vi "Dashboard Main.vi"() -> ()   [LabVIEW 2014]
uses:
  <vilib>/event_ctls.llb/eventvkey.ctl
  <vilib>/Rock Robotics/WPI/Dashboard/WPI_DashboardLogging Global.vi
  <vilib>/Utility/config.llb/Write Key (String).vi
  <vilib>/Utility/config.llb/Write Key (I32).vi
  <vilib>/Utility/config.llb/NI_LVConfig.lvlib
panel:
  out "Button 0":bool
  in  "TCP":refnum<k5>
  in  "Rec Mode":enum32{"Stop", "Record", "Playback"}(radio)
  in  "Vision":u16(ring) items=["Camera Off", "USB Camera SW", "USB Camera HW", "IP Camera"]
  out "Camera IP":string
  out "Image Message":string="Timeout in Camera Communications"
  in  "Dashboard Tab":T1(tab)
  in  "Camera Settings":T2={"Frame Rate"=30, "Compression"=30, "Size"=1} {"Frame Rate" scale=1.0..30.0; "Size" items=["640x480", "320x240", "160x120"]}
  out "MotorChart R":cluster{"Numeric":dbl, "Numeric":dbl}(graph)
  out "MotorChart L":T3(graph)
  out "MotorSliders R":cluster{"MotorSlide1":dbl, "MotorSlide2":dbl} {"MotorSlide2" scale=-1.0..1.0 scale format="%#_2e"; "MotorSlide1" scale=-1.0..1.0 scale format="%#_2e"}
  out "MotorSliders L":T4 {"MotorSlide4 2" scale=0.0..14.0 scale format="%#_2e"; "MotorSlide2" scale=-1.0..1.0 scale format="%#_2e"; "MotorSlide1" scale=-1.0..1.0 scale format="%#_2e"}
  out "Gyro":dbl(knob) scale=0.0..360.0
  out "JS1 Z":dbl(slide) scale=-1.0..1.0 scale format="%#_2e"
  out "JS1 Graph":cluster{"X":dbl, "Y":dbl}[](graph)
  out "JS1 Buttons":T5
  out "JS2 Z":dbl(slide) scale=-1.0..1.0 scale format="%#_2e"
  out "JS2 Graph":cluster{"X":dbl, "Y":dbl}[](graph)
  out "JS2 Buttons":T5
  out "Mode":T6(ring)=enum."Auto Disabled"
  in  "DB Camera Config":bool
  out "fps":dbl format="%#.1g"
  out "Mbps":dbl format="%#.1g"
  out "Mbps 2":bool
  in  "DB/String 9":string
  in  "DB/String 8":string
  in  "DB/String 7":string
  in  "DB/String 6":string
  in  "DB/String 5":string
  in  "DB/String 4":string
  in  "DB/String 3":string
  in  "DB/String 2":string
  in  "DB/String 1":string
  in  "DB/String 0":string
  in  "DB/Slider 0":dbl(slide) scale=0.0..5.0
  in  "DB/Slider 1":dbl(slide) scale=0.0..5.0
  in  "DB/Slider 2":dbl(slide) scale=0.0..5.0
  in  "DB/Slider 3":dbl(slide) scale=0.0..5.0
  out "DB/LED 3":bool
  out "DB/LED 2":bool
  out "DB/LED 1":bool
  out "DB/LED 0":bool
  in  "DB/Button 3":bool
  in  "DB/Button 2":bool
  in  "DB/Button 1":bool
  in  "DB/Button 0":bool caption="New Name"
  out "Left":dbl(knob) scale=-10.0..10.0
  out "Right":dbl(knob) scale=-10.0..10.0
  out "Inverse":bool
  out "Normal":bool
  in  "Test Slider":dbl(slide) scale=0.0..100.0 scale format="%#_3g"
  in  "On/Off":bool caption="Solenoid"
  in  "Test Name":u16(ring) items=["Select the test to run...", "Example Test", "-------------------------------", "List of tests is built in robot code.", "Replace with your own automated tests."]
  in  "Test Tree":string(tree)
  in  "Motor":cluster{"Value":dbl, "Enable":bool} {"Value" scale=-1.0..1.0 scale format="%#_3g"}
  out "Progress":T7 {"Test Progress" scale=0.0..100.0}
  in  "Rev/Fwd":cluster{"Forward":bool, "Reverse":bool}
  in  "Test Ring":u16(ring) items=["Monochrome", "Color"]
  in  "Listbox":i32(listbox)
  out "Tree":string(tree)
  out "Camera Image":T8(plugin-control)
  out "Boolean":bool
  # "Left"
  # "Front"
  # "Right"
  # "Battery"
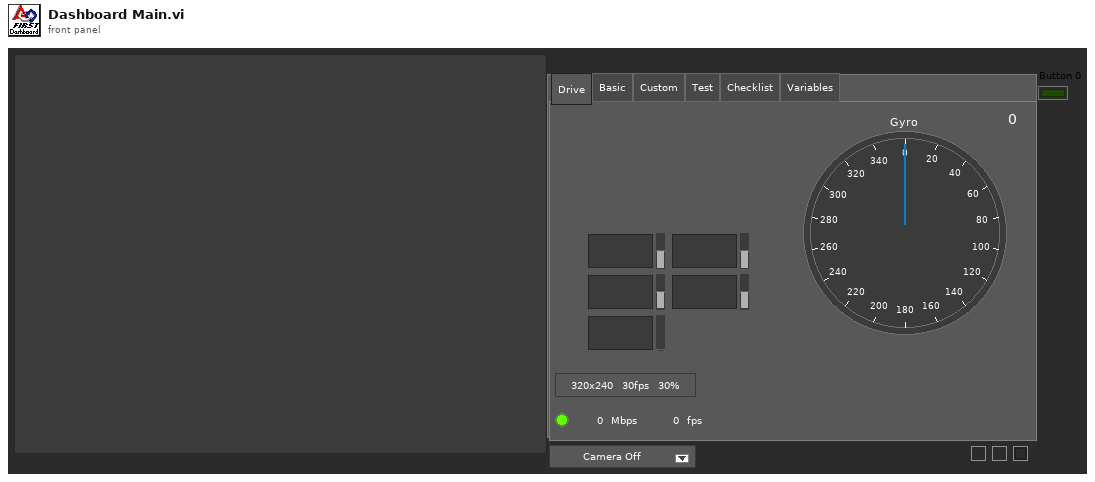
[diagram p1: front panel]
types:
  T1 = enum32{"Drive", "Basic", "Custom", "Test", "Checklist", "Variables"}
  T2 = cluster{"Frame Rate":i32, "Compression":i32, "Size":u16}
  T3 = cluster{"Numeric":dbl, "Numeric":dbl, "Battery V":dbl}
  T4 = cluster{"MotorSlide1":dbl, "MotorSlide2":dbl, "MotorSlide4 2":dbl}
  T5 = cluster{bool, bool, bool, bool, bool, bool, bool, bool, bool, bool, bool, bool}
  T6 = enum8{"Tele-Op Disabled", "Tele-Op Enabled", "Auto Disabled", "Auto Enabled", "Test Disabled", "Test Enabled", "Disconnected", "No Code", "E-Stop"}
  T7 = cluster{"Test Progress":u8, "Test Progress Text":string}
  T8 = typedef "IMAQ Image.ctl" = refnum<image>
  T9 = typedef "Image Type" = u32
  T10 = cluster{"Camera Image":refnum<vi>, "Dashboard Tab":refnum<vi>, "Boolean":refnum<vi>, "Vision":refnum<vi>, "Rec Mode":refnum<vi>, "Test Slider":refnum<vi>, "On/Off ":refnum<vi>, "Test Ring":refnum<vi>, "Rev/Fwd":refnum<vi>, "Test Name":refnum<vi>, "Motor":refnum<vi>, "Progress":refnum<vi>, "CheckList":refnum<vi>, "Tree":refnum<vi>, "Test Tree":refnum<vi>}
  T11 = typedef "NI_LVConfig.lvlib/Config Data RefNum.ctl" = refnum<k1>
  T12 = cluster{"Error Strings":string, "Disable Counts":cluster{u16, u16}, "Rail Faults":cluster{u16, u16, u16}, "Robot IP":string, "DB Mode":u8, "Event Info":cluster{"Name":string, "Type":u8, "Number":u16, "Replay":u8}, "Camera Addr":string}
  T13 = cluster{"Storage":cluster{"Disk Free":u64, "RAM Block":u32, "RAM free":u32}, "CPU Utilization":cluster{"CPU % ISR":sgl, "CPU % Time Crit":sgl, "CPU % Timed Str":sgl, "CPU % High":sgl, "CPU % Above":sgl, "CPU % Normal":sgl, "CPU % Low":sgl}, "CAN":cluster{"% Bus Utilization":sgl, "Bus Off Cnt":u32, "TX_FIFO Full Cnt":u32, "Receive Error Cnt":u8, "Transmit Error Cnt":u8}, "HID":cluster{"HID Outputs":u32, "Rumble Low":u16, "Rumble High":u16}[]}
  T14 = cluster{"Status bits":cluster{"Test Mode":bool, "Autonomous":bool, "Enabled":bool, "Code Start":bool, "Brownout":bool, "Reserved 2":bool, "Reserved 3":bool, "E-Stop":bool}, "Code Trace":cluster{"Disabled":bool, "TeleOp":bool, "Auto":bool, "Test":bool}, "Controller Type":enum16{"unknown", "cRIO", "roboRio"}, "Code?":enum16{"unknown", "noCode", "code"}, "Battery V":dbl}
  T15 = cluster{"Control Bits":cluster{"TestMode":bool, "Autonomous":bool, "Enabled":bool, "FMS Present":bool, bool, bool, bool, "E-Stop":bool}, "Team Station ":u8, "Countdown":sgl, "Joystick Values":cluster{"Axes":dbl[], "Buttons":bool[], "POVs":i16[]}[]}
  T16 = cluster{"Axes":dbl[], "Buttons":bool[], "POVs":i16[]}[]
  T17 = cluster{"Axes":dbl[], "Buttons":bool[], "POVs":i16[]}
  T18 = cluster{"Buttons[0]":bool, "Buttons[1]":bool, "Buttons[2]":bool, "Buttons[3]":bool, "Buttons[4]":bool, "Buttons[5]":bool, "Buttons[6]":bool, "Buttons[7]":bool, "Buttons[8]":bool, "Buttons[9]":bool, "Buttons[10]":bool, "Buttons[11]":bool}
  T19 = cluster{"Operation":enum16{"Update", "Clear"}, "Color Box":u32}[]
  T20 = typedef "eventvkey.ctl" = enum16{"ASCII", "Enter", "Return", "Shift", "Ctrl", "Alt", "Cmd", "Opt", "Caps", "NumLock", "Clear", "Break", "Up", "Down", "Left", "Right", "Insert", "Delete", "Home", "End", "PageUp", "PageDown", "Escape", "Help", "Pause", "ScrollLock", "F1", "F2", "F3", "F4", "F5", "F6", "F7", "F8", "F9", "F10", "F11", "F12", "F13", "F14", "F15", "F16", "F17", "F18", "F19", "F20", "F21", "F22", "F23", "F24", "Play", "VolumeUp", "VolumeDown", "Mute", "Two Byte Char"}
  T21 = cluster{"Image Size":bool, "Image Type":bool, "Pixel Value":bool, "ROI Information":bool, "Zoom Factor":bool}
  T22 = enum8{"Enabled", "Disabled", "Disabled and Grayed Out"}
  T23 = cluster{"Operation":enum16{"Update", "Clear"}, "Color Box":u32}
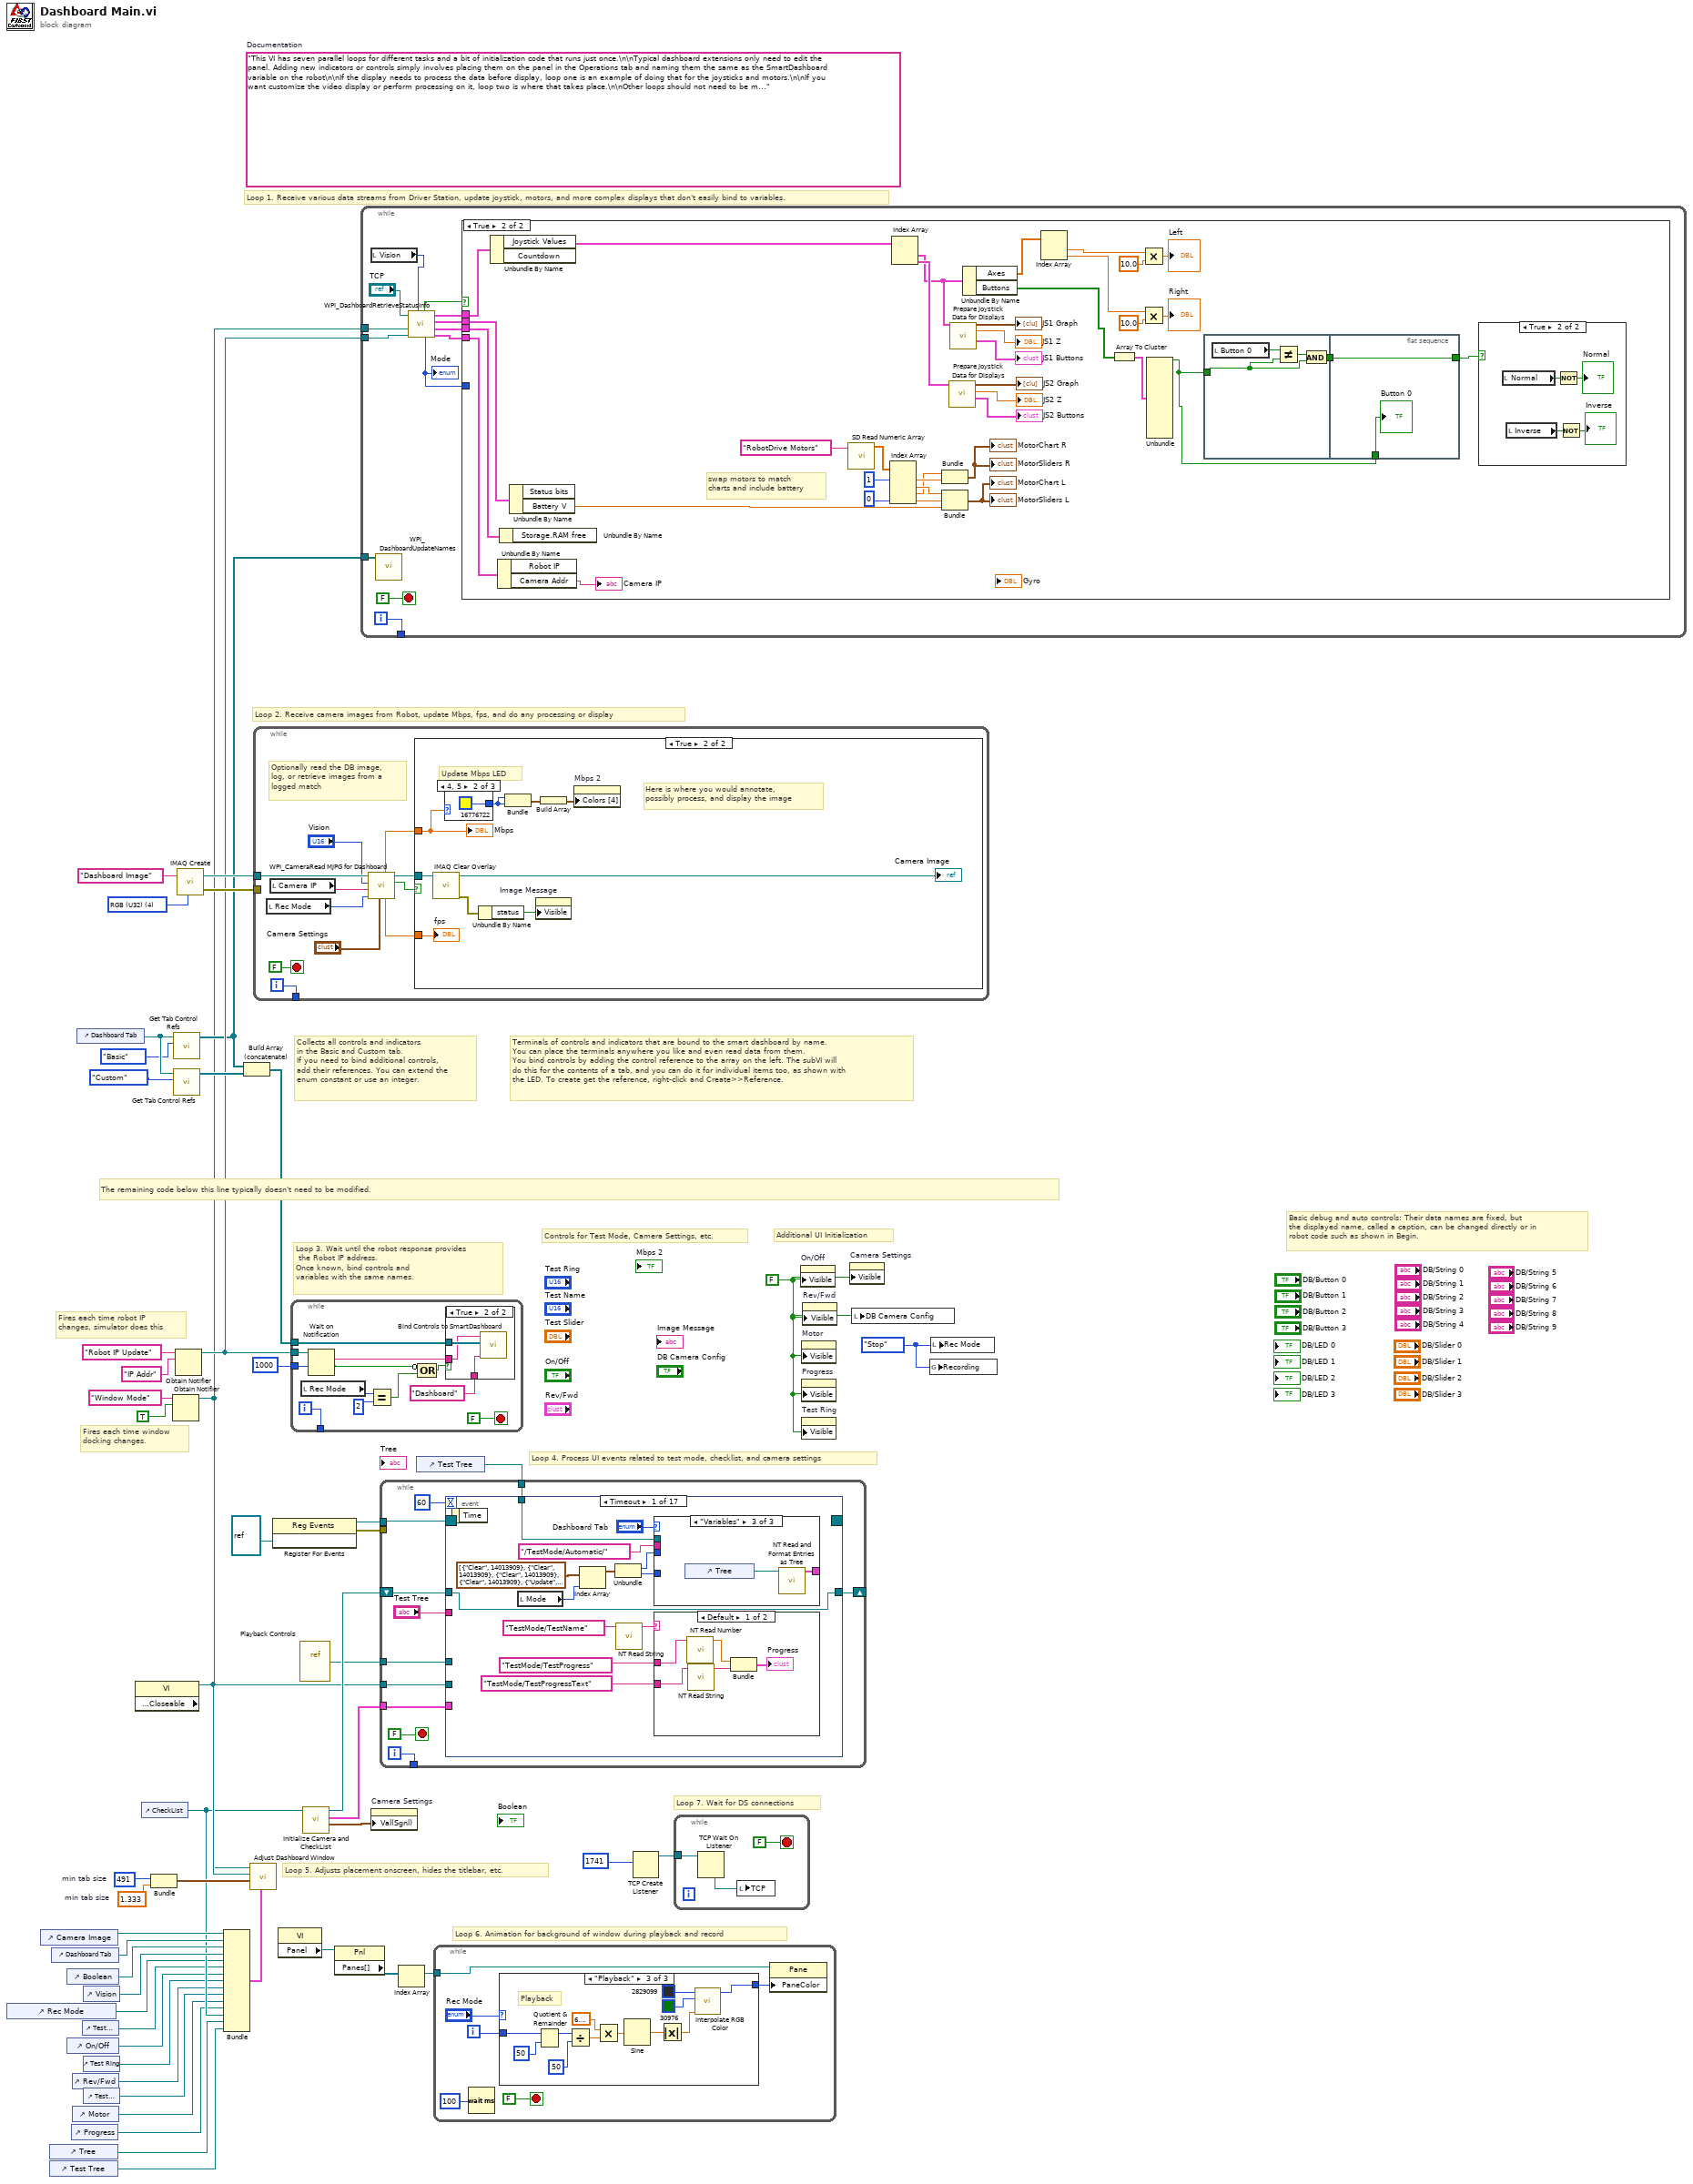
[diagram p0: block diagram]
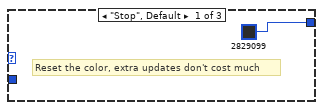
[diagram p4: hidden frame]
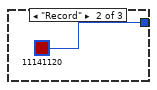
[diagram p5: hidden frame]
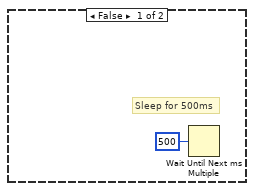
[diagram p7: hidden frame]
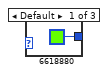
[diagram p8: hidden frame]
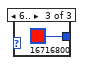
[diagram p9: hidden frame]
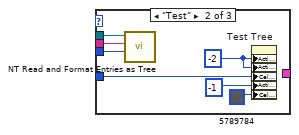
[diagram p11: hidden frame]
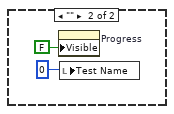
[diagram p12: hidden frame]
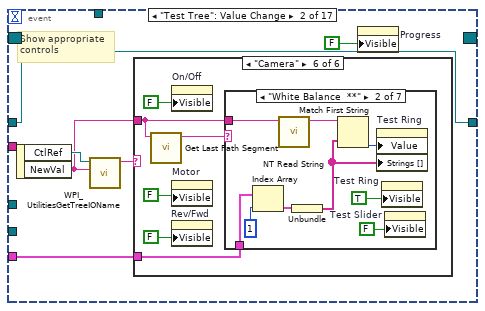
[diagram p13: hidden frame]
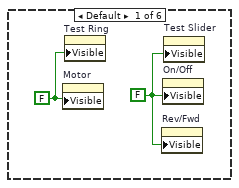
[diagram p14: hidden frame]
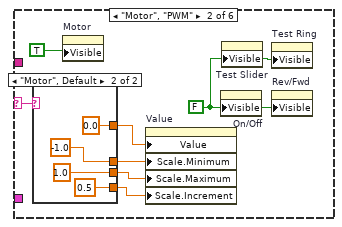
[diagram p15: hidden frame]
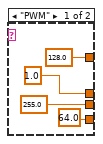
[diagram p16: hidden frame]
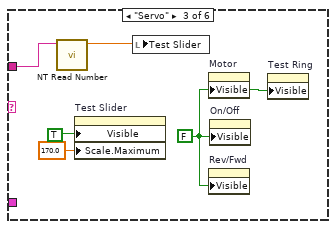
[diagram p17: hidden frame]
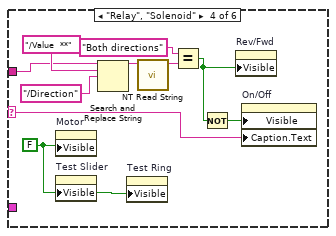
[diagram p18: hidden frame]
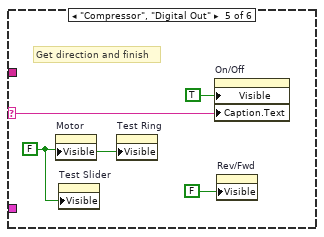
[diagram p19: hidden frame]
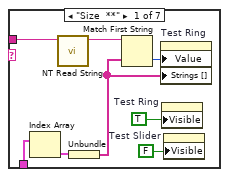
[diagram p20: hidden frame]
diagram:
  w24 = 491  # min tab size
  w23 = 1.333  # min tab size
  w32 = enum32{"Stop", "Record", "Playback"}."Stop" ("Rec Mode")
  w6 = FALSE ("Visible")
  (unwired) "This VI has seven parallel loops for different tasks and a bit of initialization code that runs just once.\n\nTypical dashboard extensions only need to edit the panel. Adding new indicators or controls simply involves placing them on the panel in the Operations tab and naming them the same as the SmartDashboard variable on the robot\n\nIf the display needs to process the data before display, loop one is an example of doing that for the joysticks and motors.\n\nIf you want customize the video display or perform processing on it, loop two is where that takes place.\n\nOther loops should not need to be modified. They are pretty standard, and document the task they perform."  # Documentation
  w52 = T9 4 items=["Grayscale (U8)", "Grayscale (I16)", "Grayscale (SGL)", "Complex (CSG)", "RGB (U32)", "HSL (U32)", "RGB (U64)"] ("Image Type")
  # "Loop 7. Wait for DS connections"
  # "Basic debug and auto controls: Their data names are fixed, but\nthe displayed name, called a caption, can be changed directly or in\nrobot code such as shown in Begin."
  # "Controls for Test Mode, Camera Settings, etc."
  # "Additional UI Initialization"
  # "Loop 6. Animation for background of window during playback and record"
  # "Fires each time robot IP\nchanges, simulator does this"
  # "Fires each time window\ndocking changes."
  # "Collects all controls and indicators\nin the Basic and Custom tab.\nIf you need to bind additional controls,\nadd their references. You can extend the\nenum constant or use an integer."
  # "The remaining code below this line typically doesn't need to be modified."
  # "Loop 4. Process UI events related to test mode, checklist, and camera settings"
  # "Terminals of controls and indicators that are bound to the smart dashboard by name.\nYou can place the terminals anywhere you like and even read data from them.\nYou bind controls by adding the control reference to the array on the left. The subVI will\ndo this for the contents of a tab, and you can do it for individual items too, as shown with\nthe LED. To create get the reference, right-click and Create>>Reference."
  # "Loop 3. Wait until the robot response provides\n the Robot IP address.\nOnce known, bind controls and\nvariables with the same names."
  # "Loop 5. Adjusts placement onscreen, hides the titlebar, etc."
  # "Loop 1. Receive various data streams from Driver Station, update joystick, motors, and more complex displays that don't easily bind to variables."
  # "Loop 2. Receive camera images from Robot, update Mbps, fps, and do any processing or display"
  n1 = control-ref of="Rec Mode"() -> (w12:refnum<vi>)
  n2 = control-ref of="Camera Image"() -> (w27:refnum<vi>)
  n3 = control-ref of="Tree"() -> (w16:refnum<vi>)
  n4 = control-ref of="Test Tree"() -> (w15:refnum<vi>)
  n5 = control-ref of="Dashboard Tab"() -> (w26:refnum<vi>)
  n6 = control-ref of="Boolean"() -> (w21:refnum<vi>)
  n7 = control-ref of="On/Off"() -> (w10:refnum<vi>)
  n8 = control-ref of="Progress"() -> (w7:refnum<vi>)
  n9 = control-ref of="Rev/Fwd"() -> (w8:refnum<vi>)
  n10 = control-ref of="Motor"() -> (w13:refnum<vi>)
  n11 = control-ref of="Dashboard Tab"() -> (w30:refnum<vi>)
  n12 = control-ref of="Test Slider"() -> (w11:refnum<vi>)
  n13 = control-ref of="Vision"() -> (w25:refnum<vi>)
  n14 = control-ref of="Test Ring"() -> (w9:refnum<vi>)
  n15 = control-ref of="Test Name"() -> (w14:refnum<vi>)
  n16 = property class="VI" props=["Front Panel.Closeable"]() -> (reference out=w31:refnum<vi>)  [unwired: 2 in, 2 out]
  n17 = control-ref of="CheckList"() -> (w17:refnum<vi>)
  n18 = Bundle("min tab size"=w24, "min tab size"=w23) -> (w22:cluster{"min tab size":i32, "min tab size":dbl})  [unwired: 1 in]
  n19 = Obtain Notifier(name (unnamed)="Window Mode", notification data type=TRUE) -> (notifier out=w3:refnum<notifier>)  [unwired: 2 in, 2 out]
  n20 = call <vilib>:"Get Tab Control Refs.vi"("Page Index"=T1."Basic" ("Dashboard Tab"), "TabControl in"=w30) -> ("ControlsOnPage"=w4:refnum<vi>[])  [unwired: 9 in]
  n21 = call <vilib>:"Get Tab Control Refs.vi"("Page Index"=T1."Custom" ("Dashboard Tab"), "TabControl in"=w30) -> ("ControlsOnPage"=w29:refnum<vi>[])  [unwired: 9 in]
  n22 = Obtain Notifier(name (unnamed)="Robot IP Update", notification data type="IP Addr" ("name (unnamed)")) -> (notifier out=w5:refnum<notifier>)  [unwired: 2 in, 2 out]
  n23 = call "IMAQ Create"("Image Name"="Dashboard Image", "Image Type"=w52) -> ("New Image"=w50:T8, "error out"=w49:errorcluster)  [unwired: 2 in, 1 out]
  n24 = Bundle("Camera Image"=w27, "Dashboard Tab"=w26, "Boolean"=w21, "Vision"=w25, "Rec Mode"=w12, "Test Slider"=w11, "On/Off"=w10, "Test Ring"=w9, "Rev/Fwd"=w8, "Test Name"=w14, "Motor"=w13, "Progress"=w7, "CheckList"=w17, "Tree"=w16, "Test Tree"=w15) -> (w18:T10)  [unwired: 1 in]
  n25 = Build Array (concatenate)(w4, w29) -> (w28:refnum<vi>[])
  n26 = call "Adjust Dashboard Window.vi"("Sizing Refnums"=w18, "Size Constraints"=w22, "VI"=w31, "Notifier in"=w3) -> ()  [unwired: 8 in]
  n27 = while {
    tunnel: w50 -> [w61]
    tunnel: w49 -> [_]
    tunnel: [w62] -> _
    i -> [w62]
    stop <- FALSE stop-if-true
    # "Optionally read the DB image,\nlog, or retrieve images from a\nlogged match"
    n28 = local read "Rec Mode"() -> (w55:enum32{"Stop", "Record", "Playback"})
    n29 = local read "Camera IP"() -> (w53:string)
    n30 = call <vilib>:"WPI_CameraRead MJPG for Dashboard.vi"("Camera Settings"="Camera Settings", "Rec Mode"=w55, "Camera IP"=w53, "Camera Mode"="Vision", "Refnum in"=w61) -> ("Active"=w59:bool, "Refnum out"=w60:T8, "FPS"=w58:dbl, "Bandwidth (Mbps)"=w57:dbl)  [unwired: 3 in]
    n31 = case shown="True" w59 {
      tunnel: w60 -> [_ w68]
      tunnel: w57 -> [_ w67]
      tunnel: w58 -> [_ w65]
      frame False {
        # "Sleep for 500ms"
        n32 = Wait Until Next ms Multiple(millisecond multiple=u32 500) -> ()  [unwired: 1 out]
      }
      frame True {
        # "Here is where you would annotate,\npossibly process, and display the image"
        # "Update Mbps LED"
        n33 = call "IMAQ Clear Overlay"("Image"=w68) -> ("error out"=w72:errorcluster, "Image Out"=→"Camera Image":T8)  [unwired: 2 in, 7 out]
        n34 = case shown="4, 5" w67 {
          tunnel: [u32 6618880 ("Color Box") u32 16776722 ("Color Box") u32 16716800 ("Color Box")] -> w69
          frame Default {
          }
          frame 4, 5 {
          }
          frame 6.. {
          }
        }
        n35 = Unbundle By Name(w72) -> ("status"=w73:bool)
        n36 = Bundle("Color Box"=w69, "Color Box"=w69) -> (w71:cluster{"Color Box":u32, "Color Box":u32})  [unwired: 1 out]
        n37 = property on="Image Message" class="Str"("Visible"=w73) -> ()  [unwired: 2 in, 2 out]
        n38 = Build Array(w71) -> (w70:cluster{"Color Box":u32, "Color Box":u32}[])
        n39 = property on="Mbps 2" class="Bool (strict)"("Colors [4]"=w70) -> ()  [unwired: 2 in, 2 out]
        "Mbps" <- w67
        "fps" <- w65
      }
    }
  }
  n40 = register-events(refnum<vi> refnum) -> (reference out=w36:refnum<event-registration>, error out=w35:errorcluster)  [unwired: 2 in]
  n41 = property class="VI"() -> ("Panel"=w39:refnum<vi>)  [unwired: 2 in, 2 out]
  n42 = while {
    tunnel: w28 -> [w88]
    tunnel: w5 -> [w86]
    tunnel: [w84] -> _
    tunnel: u32 1000 ("milliseconds to wait") -> [w83]
    i -> [w84]
    stop <- FALSE stop-if-true
    n43 = local read "Rec Mode"() -> (w79:enum32{"Stop", "Record", "Playback"})
    n44 = Wait on Notification(notifier=w86, timeout in ms (-1)=w83) -> (notification=w85:string, timed out?=w81:bool)  [unwired: 2 in, 2 out]
    n45 = Equal?(x=w79, y=u16 2 ("Rec Mode")) -> (x = y?=w80:bool)
    n46 = Compound Arithmetic op=OR(invert w81, w80) -> (w82:bool)
    n47 = case shown="True" w82 {
      tunnel: w88 -> [_ w91]
      tunnel: w85 -> [_ w90]
      tunnel: "Dashboard" -> [_ w89]
      frame False {
      }
      frame True {
        n48 = call <vilib>:"Bind Controls to SmartDashboard.vi"("Client Name"=w89, "Bound Control Refs"=w91, "Server IP Address"=w90) -> ()  [unwired: 9 in]
      }
    }
  }
  n49 = vi-ref "Playback Controls.vi"() -> (w37:refnum<vi>)
  n50 = call "Initialize Camera and CheckList.vi"("ListBox in"=w17) -> ("Cluster"=w43:cluster{"value":i32, "value":i32, "index":i32}, "Array"=w44:cluster{string[]}[], "File Refnum"=w42:T11)  [unwired: 8 in]
  n51 = property class="Pnl"(reference=w39) -> ("Panes[]"=w40:refnum<vi>[])  [unwired: 1 in, 2 out]
  n52 = while {
    tunnel: [w103] -> _
    tunnel: w5 -> [w97]
    tunnel: w4 -> [w96]
    tunnel: w3 -> [w92]
    i -> [w103]
    stop <- FALSE stop-if-true
    n53 = local read "Vision"() -> (w94:u16)
    n54 = call <vilib>:"WPI_DashboardUpdateNames.vi"("Controls on Tab"=w96) -> ()  [unwired: 11 in]
    n55 = call <vilib>:"WPI_DashboardRetrieveStatusInfo.vi"("Vision"=w94, "Binding Refnum"=w97, "Window Mode Notifier"=w92, "TCP Cnx"="TCP") -> ("Power and Errors"=w98:T12, "Robot Metrics"=w101:T13, "Status Info"=w102:T14, "Control Info"=w99:T15, "Robot Mode"=w95:T6, "Process?"=w100:bool)  [unwired: 2 in]
    "Mode" <- w95
    n56 = case shown="True" w100 {
      tunnel: w102 -> [_ w141]
      tunnel: w101 -> [_ w140]
      tunnel: w99 -> [_ w139]
      tunnel: w98 -> [_ w138]
      tunnel: w95 -> [_ _]
      frame False {
      }
      frame True {
        # "swap motors to match\ncharts and include battery"
        n57 = Unbundle By Name(w139) -> ("Joystick Values"=w126:T16)  [unwired: 1 out]
        n58 = Unbundle By Name(w138) -> ("Camera Addr"=→"Camera IP":string)  [unwired: 1 out]
        n59 = Unbundle By Name(w140) -> ()  [unwired: 1 out]
        n60 = Unbundle By Name(w141) -> ("Battery V"=w127:dbl)  [unwired: 1 out]
        n61 = call <vilib>:"SD Read Numeric Array.vi"("Name"="RobotDrive Motors") -> ("Numeric Array"=w129:dbl[])  [unwired: 8 in, 2 out]
        n62 = Index Array(array=w129, index #1=1, index #4=0) -> (element #1=w133:dbl, element #2=w134:dbl, element #3=w132:dbl, element #4=w137:dbl)  [unwired: 2 in]
        n63 = Index Array(array=w126) -> (element #1=w116:T17, element #2=w122:T17)  [unwired: 2 in]
        n64 = Bundle("Numeric"=w132, "Numeric"=w133) -> (→"MotorChart R" →"MotorSliders R":cluster{"Numeric":dbl, "Numeric":dbl})  [unwired: 1 in]
        n65 = Bundle("Numeric"=w134, "Numeric"=w137, "Battery V"=w127) -> (→"MotorChart L" →"MotorSliders L":T3)  [unwired: 1 in]
        n66 = call "Prepare Joystick Data for Displays.vi"("Joystick Values"=w122) -> ("Buttons"=→"JS2 Buttons":T18, "Z Axis"=→"JS2 Z":dbl, "Cartesian Data"=→"JS2 Graph":cluster{"X axis":dbl, "X axis":dbl}[])  [unwired: 8 in]
        n67 = call "Prepare Joystick Data for Displays.vi"("Joystick Values"=w116) -> ("Buttons"=→"JS1 Buttons":T18, "Z Axis"=→"JS1 Z":dbl, "Cartesian Data"=→"JS1 Graph":cluster{"X axis":dbl, "X axis":dbl}[])  [unwired: 8 in]
        n68 = Unbundle By Name(w116) -> ("Axes"=w117:dbl[], "Buttons"=w109:bool[])
        n69 = Index Array(array=w117) -> (element #1=w113:dbl, element #2=w110:dbl)  [unwired: 2 in]
        n70 = Array To Cluster(array=w109) -> (cluster=w108:T18)
        n71 = Multiply(x=w113, y=10.0) -> (x*y=→"Left":dbl)
        n72 = Multiply(x=w110, y=10.0) -> (x*y=→"Right":dbl)
        n73 = Unbundle(w108) -> ("Buttons[0]"=w105:bool)  [unwired: 11 out]
        n74 = flat-sequence {
          tunnel: [w143] -> w106
          tunnel: w105 -> [w142]
          tunnel: [w147] -> w107
          tunnel: w106 -> [w147]
          tunnel: w105 -> [w146]
          frame #0 {
            n75 = local read "Button 0"() -> (w145:bool)
            n76 = Not Equal?(x=w145, y=w142) -> (x != y?=w144:bool)
            n77 = And(x=w144, y=w142) -> (x .and. y?=w143:bool)
          }
          frame #1 {
            "Button 0" <- w146
          }
        }
        n78 = case shown="True" w107 {
          frame False {
          }
          frame True {
            n79 = local read "Normal"() -> (w148:bool)
            n80 = local read "Inverse"() -> (w150:bool)
            n81 = Not(x=w148) -> (.not. x?=→"Normal":bool)
            n82 = Not(x=w150) -> (.not. x?=→"Inverse":bool)
          }
        }
      }
    }
  }
  n83 = property on="Camera Settings" class="Clust (strict)"("Val(Sgnl)"=w43) -> ()  [unwired: 2 in, 2 out]
  n84 = Index Array(array=w40) -> (element=w38:refnum<vi>)  [unwired: 1 in]
  n85 = control-ref of="Test Tree"() -> (w41:refnum<vi>)
  n86 = while {
    tunnel: w44 -> [w159]
    shift-right: [w158] -> _
    shift-left: w42 -> [w157]
    tunnel: [w156] -> _
    tunnel: w41 -> [w155]
    tunnel: w37 -> [w154]
    tunnel: w36 -> [w153]
    tunnel: w35 -> [_]
    tunnel: w31 -> [w152]
    i -> [w156]
    stop <- FALSE stop-if-true
    n87 = event shown="[0] Timeout" {
      selector: w153 -> [_ _ _ _ _ _ _ _ _ _ _ _ _ _ _ _ _]
      dyn-events: [_ _ _ _ _ _ _ _ _ _ _ _ _ w397 _ _ _] -> _
      timeout: u32 60 ("milliseconds to wait") -> [_ _ _ _ _ _ _ _ _ _ _ _ _ _ _ _ _]
      tunnel: w155 -> [w171 _ _ _ _ _ _ _ _ _ _ _ _ _ _ _ _]
      tunnel: "Test Tree" -> [_ _ _ _ _ _ _ _ w366 w374 w376 w380 w388 _ _ _ _]
      tunnel: w159 -> [_ w193 _ _ _ _ w330 w360 _ _ _ _ _ _ _ _ _]
      tunnel: [w167 w192 w291 w296 w304 w316 w329 w353 w365 w372 w375 w379 w387 w399 w413 w414 w424] -> w158
      tunnel: w157 -> [w167 w192 w291 w296 w304 w316 w328 w353 w365 w372 w375 w379 w387 w399 w413 w414 w424]
      tunnel: w154 -> [_ _ _ _ _ _ _ _ _ _ _ _ _ w400 _ w417 _]
      tunnel: w152 -> [_ _ _ _ _ _ _ _ _ _ _ _ _ w395 _ _ _]
      event Timeout {
        n88 = event-data() -> ()  [unwired: 1 in, 1 out]
        n89 = local read "Mode"() -> (w170:T6)
        n90 = Index Array(array=T19 [{"Operation"=enum."Clear", "Color Box"=14013909}, {"Operation"=enum."Clear", "Color Box"=14013909}, {"Operation"=enum."Clear", "Color Box"=14013909}, {"Operation"=enum."Clear", "Color Box"=14013909}, {"Operation"=enum."Update", "Color Box"=14013909}, {"Operation"=enum."Update", "Color Box"=16777215}, {"Operation"=enum."Clear", "Color Box"=14013909}, {"Operation"=enum."Clear", "Color Box"=14013909}, {"Operation"=enum."Clear", "Color Box"=14013909}], index=w170) -> (element=w165:T23)
        n91 = Unbundle(w165) -> ("Operation"=w164:enum16{"Update", "Clear"}, "Color Box"=w163:u32)
        n92 = call <vilib>:"NT Read String.vi"("Name"="TestMode/TestName") -> ("String"=w174:string)  [unwired: 9 in, 1 out]
        n93 = case shown="\"Variables\"" "Dashboard Tab" {
          tunnel: w171 -> [_ w182 _]
          tunnel: "/TestMode/Automatic/" ("Name Pattern") -> [_ w181 _]
          tunnel: w164 -> [_ w180 _]
          tunnel: [_ _ w184] -> _
          tunnel: w163 -> [_ w176 _]
          frame "Custom", Default {
          }
          frame "Test" {
            w179 = -2 ("Active Item:Row Number")
            n94 = call <vilib>:"NT Read and Format Entries as Tree.vi"("Operation"=w180, "Name Pattern"=w181, "Tree Refnum"=w182) -> ()  [unwired: 7 in, 2 out]
            n95 = property on="Test Tree" class="Tree (strict)"("Active Item Row Number"=w179, "ActiveColNum"=w179, "CellBG"=w176, "Active Item Row Number"=-1 ("Active Item:Row Number"), "CellBG"=u32 5789784 ("Color Box")) -> ()  [unwired: 2 in, 2 out]
          }
          frame "Variables" {
            n96 = control-ref of="Tree"() -> (w183:refnum<vi>)
            n97 = call <vilib>:"NT Read and Format Entries as Tree.vi"("Tree Refnum"=w183) -> ("Formatted Strings"=w184:cluster{"Name":string, "Value":string}[])  [unwired: 9 in, 1 out]
          }
        }
        n98 = case shown="Default" w174 {
          tunnel: "TestMode/TestProgress" ("Name") -> [w186 _]
          tunnel: "TestMode/TestProgressText" ("Name") -> [w185 _]
          frame Default {
            n99 = call <vilib>:"NT Read Number.vi"("Name"=w186) -> ("Numeric"=w187:dbl)  [unwired: 9 in, 1 out]
            n100 = call <vilib>:"NT Read String.vi"("Name"=w185) -> ("String"=w188:string)  [unwired: 9 in, 1 out]
            n101 = Bundle("Numeric"=w187, "String"=w188) -> (→"Progress":cluster{"Numeric":dbl, "String":string})  [unwired: 1 in]
          }
          frame "" {
            n102 = property on="Progress" class="Clust (strict)"("Visible"=FALSE) -> ()  [unwired: 2 in, 2 out]
            n103 = local write "Test Name"(u16 0) -> ()
          }
        }
      }
      event "Test Tree": Value Change {
        # "Show appropriate\ncontrols"
        n104 = event-data() -> ("CtlRef"=w196:refnum<vi>, "NewVal"=w194:string)  [unwired: 1 in]
        n105 = call <vilib>:"WPI_UtilitiesGetTreeIOName.vi"("NewVal"=w194, "TreeControl in"=w196) -> ("I/O Name"=w197:string)  [unwired: 9 in]
        n106 = case shown="\"Camera\"" w197 {
          selector: w197 -> [_ w204 _ w222 w231 _]
          tunnel: w194 -> [_ _ w219 w221 _ w238]
          tunnel: w193 -> [_ _ _ _ _ w237]
          frame Default {
            w199 = FALSE ("Visible")
            w198 = FALSE ("Visible")
            n107 = property on="Motor" class="Clust (strict)"("Visible"=w198) -> ()  [unwired: 2 in, 2 out]
            n108 = property on="Test Ring" class="Ring (strict)"("Visible"=w198) -> ()  [unwired: 2 in, 2 out]
            n109 = property on="Rev/Fwd" class="Clust (strict)"("Visible"=w199) -> ()  [unwired: 2 in, 2 out]
            n110 = property on="On/Off" class="Bool (strict)"("Visible"=w199) -> ()  [unwired: 2 in, 2 out]
            n111 = property on="Test Slider" class="Slide (strict)"("Visible"=w199) -> ()  [unwired: 2 in, 2 out]
          }
          frame "Motor", "PWM" {
            w205 = FALSE ("Visible")
            n112 = case shown="\"Motor\", Default" w204 {
              tunnel: [1.0 ("Value") -1.0 ("Value")] -> w203
              tunnel: [255.0 ("Value") 1.0 ("Value")] -> w202
              tunnel: [128.0 ("Value") 0.0 ("Value")] -> w201
              tunnel: [64.0 ("Value") 0.5 ("Value")] -> w200
              frame "PWM" {
              }
              frame "Motor", Default {
              }
            }
            n113 = property on="Motor" class="Clust (strict)"("Visible"=TRUE) -> ()  [unwired: 2 in, 2 out]
            n114 = property on="Value" class="Slide (strict)"("Value"=w201, "Scale.Minimum"=w203, "Scale.Maximum"=w202, "Scale.Increment"=w200) -> ()  [unwired: 2 in, 2 out]
            n115 = property on="On/Off" class="Bool (strict)"("Visible"=w205) -> ()  [unwired: 2 in, 2 out]
            n116 = property on="Test Slider" class="Slide (strict)"("Visible"=w205) -> ()  [unwired: 2 in, 2 out]
            n117 = property on="Test Ring" class="Ring (strict)"("Visible"=w205) -> ()  [unwired: 2 in, 2 out]
            n118 = property on="Rev/Fwd" class="Clust (strict)"("Visible"=w205) -> ()  [unwired: 2 in, 2 out]
          }
          frame "Servo" {
            w217 = FALSE ("Visible")
            n119 = call <vilib>:"NT Read Number.vi"("Name"=w219) -> ("Numeric"=w218:dbl)  [unwired: 9 in, 1 out]
            n120 = property on="Test Slider" class="Slide (strict)"("Visible"=TRUE, "Scale.Maximum"=170.0 ("Scale.Range:Maximum")) -> ()  [unwired: 2 in, 2 out]
            n121 = local write "Test Slider"(w218) -> ()
            n122 = property on="Motor" class="Clust (strict)"("Visible"=w217) -> ()  [unwired: 2 in, 2 out]
            n123 = property on="Rev/Fwd" class="Clust (strict)"("Visible"=w217) -> ()  [unwired: 2 in, 2 out]
            n124 = property on="On/Off" class="Bool (strict)"("Visible"=w217) -> ()  [unwired: 2 in, 2 out]
            n125 = property on="Test Ring" class="Ring (strict)"("Visible"=w217) -> ()  [unwired: 2 in, 2 out]
          }
          frame "Relay", "Solenoid" {
            w220 = FALSE ("Visible")
            n126 = property on="Motor" class="Clust (strict)"("Visible"=w220) -> ()  [unwired: 2 in, 2 out]
            n127 = property on="Test Slider" class="Slide (strict)"("Visible"=w220) -> ()  [unwired: 2 in, 2 out]
            n128 = Search and Replace String(input string=w221, search string="/Value  **", replace string="/Direction") -> (result string=w227:string)  [unwired: 5 in, 3 out]
            n129 = property on="Test Ring" class="Ring (strict)"("Visible"=w220) -> ()  [unwired: 2 in, 2 out]
            n130 = call <vilib>:"NT Read String.vi"("Name"=w227) -> ("String"=w225:string)  [unwired: 9 in, 1 out]
            n131 = Equal?(x="Both directions", y=w225) -> (x = y?=w223:bool)
            n132 = Not(x=w223) -> (.not. x?=w224:bool)
            n133 = property on="Rev/Fwd" class="Clust (strict)"("Visible"=w223) -> ()  [unwired: 2 in, 2 out]
            n134 = property on="On/Off" class="Bool (strict)"("Visible"=w224, "Caption.Text"=w222) -> ()  [unwired: 2 in, 2 out]
          }
          frame "Compressor", "Digital Out" {
            w230 = FALSE ("Visible")
            # "Get direction and finish"
            n135 = property on="Motor" class="Clust (strict)"("Visible"=w230) -> ()  [unwired: 2 in, 2 out]
            n136 = property on="Test Slider" class="Slide (strict)"("Visible"=w230) -> ()  [unwired: 2 in, 2 out]
            n137 = property on="Test Ring" class="Ring (strict)"("Visible"=w230) -> ()  [unwired: 2 in, 2 out]
            n138 = property on="On/Off" class="Bool (strict)"("Visible"=TRUE, "Caption.Text"=w231) -> ()  [unwired: 2 in, 2 out]
            n139 = property on="Rev/Fwd" class="Clust (strict)"("Visible"=FALSE) -> ()  [unwired: 2 in, 2 out]
          }
          frame "Camera" {
            n140 = call <vilib>:"Get Last Path Segment.vi"("String in"=w238) -> ("String out"=w239:string)  [unwired: 10 in]
            n141 = property on="On/Off" class="Bool (strict)"("Visible"=FALSE) -> ()  [unwired: 2 in, 2 out]
            n142 = property on="Motor" class="Clust (strict)"("Visible"=FALSE) -> ()  [unwired: 2 in, 2 out]
            n143 = property on="Rev/Fwd" class="Clust (strict)"("Visible"=FALSE) -> ()  [unwired: 2 in, 2 out]
            n144 = case shown="\"White Balance  **\"" w239 {
              tunnel: w238 -> [w245 w254 w263 w272 w281 _ w287]
              tunnel: w237 -> [w243 w251 w260 w269 w278 _ _]
              frame "Size  **" {
                n145 = Index Array(array=w243) -> (element=w242:cluster{string[]})  [unwired: 1 in]
                n146 = call <vilib>:"NT Read String.vi"("Name"=w245) -> ("String"=w244:string)  [unwired: 9 in, 1 out]
                n147 = Unbundle(w242) -> (w240:string[])
                n148 = Match First String(2:w240, 3:w244) -> (0:w241:i32)  [unwired: 1 out]
                n149 = property on="Test Ring" class="Ring (strict)"("Value"=w241, "Strings []"=w240) -> ()  [unwired: 2 in, 2 out]
                n150 = property on="Test Ring" class="Ring (strict)"("Visible"=TRUE) -> ()  [unwired: 2 in, 2 out]
                n151 = property on="Test Slider" class="Slide (strict)"("Visible"=FALSE) -> ()  [unwired: 2 in, 2 out]
              }
              frame "White Balance  **" {
                n152 = Index Array(array=w251, index=1) -> (element=w252:cluster{string[]})
                n153 = call <vilib>:"NT Read String.vi"("Name"=w254) -> ("String"=w253:string)  [unwired: 9 in, 1 out]
                n154 = Unbundle(w252) -> (w249:string[])
                n155 = Match First String(2:w249, 3:w253) -> (0:w248:i32)  [unwired: 1 out]
                n156 = property on="Test Ring" class="Ring (strict)"("Value"=w248, "Strings []"=w249) -> ()  [unwired: 2 in, 2 out]
                n157 = property on="Test Ring" class="Ring (strict)"("Visible"=TRUE) -> ()  [unwired: 2 in, 2 out]
                n158 = property on="Test Slider" class="Slide (strict)"("Visible"=FALSE) -> ()  [unwired: 2 in, 2 out]
              }
              frame "Exposure  **" {
                n159 = Index Array(array=w260, index=2) -> (element=w261:cluster{string[]})
                n160 = call <vilib>:"NT Read String.vi"("Name"=w263) -> ("String"=w262:string)  [unwired: 9 in, 1 out]
                n161 = Unbundle(w261) -> (w257:string[])
                n162 = Match First String(2:w257, 3:w262) -> (0:w258:i32)  [unwired: 1 out]
                n163 = property on="Test Ring" class="Ring (strict)"("Value"=w258, "Strings []"=w257) -> ()  [unwired: 2 in, 2 out]
                n164 = property on="Test Ring" class="Ring (strict)"("Visible"=TRUE) -> ()  [unwired: 2 in, 2 out]
                n165 = property on="Test Slider" class="Slide (strict)"("Visible"=FALSE) -> ()  [unwired: 2 in, 2 out]
              }
              frame "Exposure Priority  **" {
                n166 = Index Array(array=w269, index=3) -> (element=w270:cluster{string[]})
                n167 = call <vilib>:"NT Read String.vi"("Name"=w272) -> ("String"=w271:string)  [unwired: 9 in, 1 out]
                n168 = Unbundle(w270) -> (w266:string[])
                n169 = Match First String(2:w266, 3:w271) -> (0:w267:i32)  [unwired: 1 out]
                n170 = property on="Test Ring" class="Ring (strict)"("Value"=w267, "Strings []"=w266) -> ()  [unwired: 2 in, 2 out]
                n171 = property on="Test Ring" class="Ring (strict)"("Visible"=TRUE) -> ()  [unwired: 2 in, 2 out]
                n172 = property on="Test Slider" class="Slide (strict)"("Visible"=FALSE) -> ()  [unwired: 2 in, 2 out]
              }
              frame "Color Enable  **" {
                n173 = Index Array(array=w278, index=4) -> (element=w279:cluster{string[]})
                n174 = call <vilib>:"NT Read String.vi"("Name"=w281) -> ("String"=w280:string)  [unwired: 9 in, 1 out]
                n175 = Unbundle(w279) -> (w275:string[])
                n176 = Match First String(2:w275, 3:w280) -> (0:w276:i32)  [unwired: 1 out]
                n177 = property on="Test Ring" class="Ring (strict)"("Value"=w276, "Strings []"=w275) -> ()  [unwired: 2 in, 2 out]
                n178 = property on="Test Ring" class="Ring (strict)"("Visible"=TRUE) -> ()  [unwired: 2 in, 2 out]
                n179 = property on="Test Slider" class="Slide (strict)"("Visible"=FALSE) -> ()  [unwired: 2 in, 2 out]
              }
              frame Default {
                n180 = property on="Test Ring" class="Ring (strict)"("Visible"=FALSE) -> ()  [unwired: 2 in, 2 out]
                n181 = property on="Test Slider" class="Slide (strict)"("Visible"=FALSE) -> ()  [unwired: 2 in, 2 out]
              }
              frame "Brightness  **", "Color Level  **", "Compression  **", "FPS  **", "Sharpness  **" {
                n182 = call <vilib>:"NT Read Number.vi"("Name"=w287) -> ("Numeric"=w286:dbl)  [unwired: 9 in, 1 out]
                n183 = local write "Test Slider"(w286) -> ()
                n184 = property on="Test Slider" class="Slide (strict)"("Visible"=TRUE, "Scale.Maximum"=100.0 ("Scale.Range:Maximum")) -> ()  [unwired: 2 in, 2 out]
                n185 = property on="Test Ring" class="Ring (strict)"("Visible"=FALSE) -> ()  [unwired: 2 in, 2 out]
              }
            }
          }
        }
        n186 = property on="Progress" class="Clust (strict)"("Visible"=FALSE) -> ()  [unwired: 2 in, 2 out]
      }
      event "Test Name": Mouse Enter {
        # "Populate the ring with the list of tests"
        n187 = event-data() -> ()  [unwired: 1 in, 1 out]
        n188 = call <vilib>:"NT Read String Array.vi"("Name"="TestMode/TestList") -> ("String Array"=w295:string[])  [unwired: 9 in, 1 out]
        n189 = Build Array (concatenate)("Select the test to run...", w295) -> (w294:string[])
        n190 = property on="Test Name" class="Ring (strict)"("Strings []"=w294) -> ()  [unwired: 2 in, 2 out]
      }
      event "Test Name": Value Change {
        w297 = FALSE ("Visible")
        # "Tell the robot the test name to run"
        n191 = event-data() -> ("NewVal"=w301:u16)  [unwired: 1 in]
        n192 = property on="Test Name" class="Ring (strict)"() -> ("Strings []"=w302:string[])  [unwired: 2 in, 2 out]
        n193 = local write "Progress"(T7 {"Test Progress"=0, "Test Progress Text"=""} ("Progress")) -> ()
        n194 = Index Array(array=w302, index=w301) -> (element=w300:string)
        n195 = call <vilib>:"NT Write String.vi"("String"=w300, "Name"="TestMode/TestName") -> ()  [unwired: 9 in, 1 out]
        n196 = property on="Progress" class="Clust (strict)"("Visible"=TRUE) -> ()  [unwired: 2 in, 2 out]
        n197 = property on="Motor" class="Clust (strict)"("Visible"=w297) -> ()  [unwired: 2 in, 2 out]
        n198 = property on="Test Slider" class="Slide (strict)"("Visible"=w297) -> ()  [unwired: 2 in, 2 out]
        n199 = property on="On/Off" class="Bool (strict)"("Visible"=w297) -> ()  [unwired: 2 in, 2 out]
        n200 = property on="Rev/Fwd" class="Clust (strict)"("Visible"=w297) -> ()  [unwired: 2 in, 2 out]
        n201 = property on="Test Ring" class="Ring (strict)"("Visible"=w297) -> ()  [unwired: 2 in, 2 out]
      }
      event "Listbox": Double Click {
        # "Shift clears all"
        # "Update symbols on the listbox"
        n202 = event-data() -> ("PlatMods.Shift"=w305:bool, "Row"=w307:i32)  [unwired: 1 in]
        n203 = case shown="True" w305 {
          tunnel: w307 -> [w311 _]
          tunnel: 1 -> [w310 _]
          frame False {
            n204 = property on="Listbox" class="LstBox (strict)"() -> ("Item Symbols"=w309:i32[])  [unwired: 2 in, 2 out]
            n205 = Replace Array Subset(array=w309, new element=w310, index=w311) -> (w308:i32[])
            n206 = property on="Listbox" class="LstBox (strict)"("Item Symbols"=w308) -> ()  [unwired: 2 in, 2 out]
          }
          frame True {
            w312 = 0 ("Top Row")
            n207 = property on="Listbox" class="LstBox (strict)"() -> ("Number of Rows"=w314:u32)  [unwired: 2 in, 2 out]
            n208 = Initialize Array(0, w314) -> (w313:i32[])
            n209 = property on="Listbox" class="LstBox (strict)"("Top Row"=w312, "Value"=w312, "Item Symbols"=w313) -> ()  [unwired: 2 in, 2 out]
          }
        }
      }
      event "Listbox": Key Down {
        # "Update symbols on the listbox\nLeft and right keys check and uncheck"
        n210 = event-data() -> ("VKey"=w318:T20)  [unwired: 1 in]
        n211 = case shown="\"Left\", \"Right\"" w318 {
          selector: w318 -> [w323 _]
          tunnel: eventvkey."Left" ("VKey") -> [w321 _]
          frame "Left", "Right" {
            n212 = Equal?(x=w321, y=w323) -> (x = y?=w322:bool)
            n213 = Select(t=0, s=w322, f=1) -> (s? t:f=w324:i32)
            n214 = property on="Listbox" class="LstBox (strict)"() -> ("Item Symbols"=w327:i32[])  [unwired: 2 in, 2 out]
            n215 = Replace Array Subset(array=w327, new element=w324, index="Listbox") -> (w326:i32[])
            n216 = property on="Listbox" class="LstBox (strict)"("Item Symbols"=w326) -> ()  [unwired: 2 in, 2 out]
          }
          frame Default {
          }
        }
      }
      event "DB Camera Config": Value Change {
        # "Show or hide the cluster of controls, store in ini file"
        n217 = event-data() -> ("NewVal"=w331:bool)  [unwired: 1 in]
        n218 = case shown="False" w331 {
          tunnel: w330 -> [w340 _]
          tunnel: [w333 w351] -> w329
          tunnel: w328 -> [w332 w351]
          frame False {
            w347 = "Camera"
            w350 = FALSE ("Visible")
            n219 = local read "Camera Settings"() -> (w339:T2)
            n220 = Index Array(array=w340) -> (element=w343:cluster{string[]})  [unwired: 1 in]
            n221 = Unbundle(w339) -> ("Frame Rate"=w338:i32, "Compression"=w337:i32, "Size"=w341:u16)
            n222 = Unbundle(w343) -> (w342:string[])
            n223 = Index Array(array=w342, index=w341) -> (element=w336:string)
            n224 = call-poly <vilib>:"Write Key.vi"("section"=w347, "value"=w336, "key"="Size", "refnum"=w332) -> ("refnum out"=w349:T11)  [unwired: 2 in, 5 out]
            n225 = call-poly <vilib>:"Write Key.vi"("section"=w347, "value"=w338, "key"="FrameRate", "refnum"=w349) -> ("refnum out"=w348:T11)  [unwired: 1 in, 6 out]
            n226 = property on="Camera Settings" class="Clust (strict)"("Visible"=w350) -> ()  [unwired: 2 in, 2 out]
            n227 = local write "DB Camera Config"(w350) -> ()
            n228 = call-poly <vilib>:"Write Key.vi"("section"=w347, "value"=w337, "key"="Compression", "refnum"=w348) -> ("refnum out"=w334:T11)  [unwired: 1 in, 6 out]
            n229 = call <vilib>:"Close Config Data.vi"("refnum"=w334) -> ("file path"=w335:path)  [unwired: 2 in, 8 out]
            n230 = call <vilib>:"Open Config Data.vi"("configuration file path"=w335) -> ("refnum"=w333:T11)  [unwired: 8 in, 2 out]
          }
          frame True {
            n231 = property on="Camera Settings" class="Clust (strict)"("Visible"=TRUE) -> ()  [unwired: 2 in, 2 out]
          }
        }
      }
      event "Camera Settings": Value Change {
        # "Update summary string when any elements of DB camera change"
        n232 = event-data() -> ("NewVal"=w364:T2)  [unwired: 1 in]
        n233 = Index Array(array=w360) -> (element=w359:cluster{string[]})  [unwired: 1 in]
        n234 = Unbundle(w364) -> ("Frame Rate"=w355:i32, "Compression"=w354:i32, "Size"=w357:u16)
        n235 = Unbundle(w359) -> (w358:string[])
        n236 = Index Array(array=w358, index=w357) -> (element=w356:string)
        n237 = Format Into String(format string="%s   %dfps   %d%%", w356, w355, w354) -> (resulting string=w361:string)  [unwired: 2 in, 1 out]
        n238 = Build Array(w361) -> (w362:string[])
        n239 = property on="DB Camera Config" class="Bool (strict)"("Strings [4]"=w362) -> ()  [unwired: 2 in, 2 out]
      }
      event "Motor.Enable": Value Change {
        # "When the test mode otor enable helper is set, update that\ntree row item's value"
        n240 = event-data() -> ("NewVal"=w370:bool)  [unwired: 1 in]
        n241 = Unbundle("Motor") -> ("Value"=w369:dbl)  [unwired: 1 out]
        n242 = Select(t=w369, s=w370, f=0.0) -> (s? t:f=w367:dbl)
        n243 = call <vilib>:"NT Write Number.vi"("Numeric"=w367, "Name"=w366) -> ()  [unwired: 9 in, 1 out]
      }
      event "Test Slider": Value Change {
        # "When the test mode slider helper is set, update that\ntree row item's value"
        n244 = event-data() -> ("NewVal"=w373:dbl)  [unwired: 1 in]
        n245 = call <vilib>:"NT Write Number.vi"("Numeric"=w373, "Name"=w374) -> ()  [unwired: 9 in, 1 out]
      }
      event "On/Off": Value Change {
        # "When the test mode on/off helper value is set, update that\ntree row item's value"
        n246 = event-data() -> ("NewVal"=w378:bool)  [unwired: 1 in]
        n247 = Boolean To (0,1)(Boolean=w378) -> (0, 1=w377:i16)
        n248 = call <vilib>:"NT Write Number.vi"("Numeric"=w377, "Name"=w376) -> ()  [unwired: 9 in, 1 out]
      }
      event "Rev/Fwd": Value Change {
        # "When the test mode helper value for relays is set, update that\ntree row item's value"
        n249 = event-data() -> ("NewVal.Forward"=w386:bool, "NewVal.Reverse"=w385:bool)  [unwired: 1 in]
        n250 = Boolean To (0,1)(Boolean=w386) -> (0, 1=w382:i16)
        n251 = Boolean To (0,1)(Boolean=w385) -> (0, 1=w384:i16)
        n252 = Negate(x=w384) -> (-x=w383:i16)
        n253 = Add(x=w382, y=w383) -> (x+y=w381:i16)
        n254 = call <vilib>:"NT Write Number.vi"("Numeric"=w381, "Name"=w380) -> ()  [unwired: 9 in, 1 out]
      }
      event "Test Ring": Value Change {
        # "When a test mode helper value is selected from the ring,\nset the tree item's variable to the string value"
        n255 = event-data() -> ("NewVal"=w390:u16)  [unwired: 1 in]
        n256 = property on="Test Ring" class="Ring (strict)"() -> ("Strings []"=w391:string[])  [unwired: 2 in, 2 out]
        n257 = Index Array(array=w391, index=w390) -> (element=w389:string)
        n258 = call <vilib>:"NT Write String.vi"("String"=w389, "Name"=w388) -> ()  [unwired: 9 in, 1 out]
      }
      event "Rec Mode": Value Change {
        # "Update globals for recording mode and path to read log from.\nClear when logging and let NetworkTables set path for vision to\nuse."
        n259 = event-data() -> ("NewVal"=w401:enum32{"Stop", "Record", "Playback"})  [unwired: 1 in]
        n260 = global write "WPI_DashboardLogging Global.vi" "Logging Filename"(path "") -> ()
        n261 = case shown="\"Playback\"" w401 {
          tunnel: w400 -> [_ w403 w411]
          tunnel: [_ _ w410] -> w397
          tunnel: [_ _ w409] -> _
          tunnel: w395 -> [_ _ w407]
          tunnel: cluster{i32, i32} {-250, 170} -> [_ _ w406]
          tunnel: [_ _ T21 {"Image Size"=TRUE, "Image Type"=TRUE, "Pixel Value"=TRUE, "ROI Information"=TRUE, "Zoom Factor"=FALSE} ("Image Information Shown:All Elements")] -> w393
          tunnel: [_ _ TRUE ("Zoom Factor")] -> w392
          frame Default {
          }
          frame "Stop", "Record" {
            # "Place Window too"
            n262 = invoke class="VI" method="FP.Close"(reference=w403) -> (reference out=w402:refnum<vi>)  [unwired: 2 in, 2 out]
            n263 = invoke class="VI" method="Abort VI"(reference=w402) -> ()  [unwired: 2 in, 3 out]
          }
          frame "Playback" {
            n264 = call "Open Playback Panel.vi"("Offset"=w406, "DB VI Ref"=w407, "Playback in"=w411) -> ("Playback out"=w408:refnum<vi>)  [unwired: 8 in]
            n265 = register-events(w408) -> (reference out=w410:refnum<event-registration>, error out=w409:errorcluster)  [unwired: 2 in]
          }
        }
        n266 = global write "WPI_DashboardLogging Global.vi" "Recording"(w401) -> ()
        n267 = property on="Camera Image" class="ImageControl"("Image Information Shown"=w393, "Image Information Visible"=w392) -> ()  [unwired: 2 in, 2 out]
        n268 = call <vilib>:"WPI_DashboardNT Log FieldName Cache.vi"("Operation"=enum16{"Lookup/Add", "Index", "Clear"}."Clear") -> ()  [unwired: 8 in, 3 out]
      }
      event Panel Close {
        w412 = enum32{"Stop", "Record", "Playback"}."Stop" ("Rec Mode")
        # "Playback window has been closed, abort"
        n269 = event-data() -> ()  [unwired: 1 in, 4 out]
        n270 = local write "Rec Mode"(w412) -> ()
        n271 = global write "WPI_DashboardLogging Global.vi" "Recording"(w412) -> ()
      }
      event Panel Close {
        # "Abort playback window and ourself"
        n272 = event-data() -> ()  [unwired: 1 in, 4 out]
        n273 = invoke class="VI" method="FP.Close"(reference=w417) -> (reference out=w416:refnum<vi>)  [unwired: 2 in, 2 out]
        n274 = invoke class="VI" method="Abort VI"(reference=w416) -> (error out=w415:errorcluster)  [unwired: 2 in, 2 out]
        n275 = invoke class="VI" method="Abort VI"(error in=w415) -> ()  [unwired: 2 in, 3 out]
      }
      event "Vision": Value Change {
        # "Enable/Disable Compression slider.\nHW USB is hard-coded into the camera"
        n276 = event-data() -> ("NewVal"=w423:u16)  [unwired: 1 in]
        n277 = Equal?(x=w423, y=u32 2 ("milliseconds to wait")) -> (x = y?=w421:bool)
        n278 = Select(t=T22."Disabled and Grayed Out" ("Disabled"), s=w421, f=T22."Enabled" ("Disabled")) -> (s? t:f=w418:T22)
        n279 = property on="Compression" class="Slide (strict)"("DisabledEnum"=w418) -> ()  [unwired: 2 in, 2 out]
      }
    }
  }
  n280 = while {
    tunnel: w38 -> [w426]
    i -> [w429]
    stop <- FALSE stop-if-true
    n281 = Wait (ms)(milliseconds to wait=u32 100) -> ()  [unwired: 1 out]
    n282 = case shown="\"Playback\"" "Rec Mode" {
      tunnel: w429 -> [_ _ w444]
      tunnel: [u32 2829099 ("Base Color") u32 11141120 ("Target Color") w433] -> w425
      frame "Stop", Default {
        # "Reset the color, extra updates don't cost much"
      }
      frame "Record" {
      }
      frame "Playback" {
        # "Playback"
        n283 = Quotient & Remainder(x=w444, y=u32 50 ("milliseconds to wait")) -> (x-y*floor(x/y)=w440:u32)  [unwired: 1 out]
        n284 = Divide(x=w440, y=u32 50 ("milliseconds to wait")) -> (x/y=w437:dbl)
        n285 = Multiply(x=6.283185307179586, y=w437) -> (x*y=w442:dbl)
        n286 = Sine(x=w442) -> (sin(x)=w441:dbl)
        n287 = Absolute Value(x=w441) -> (abs(x)=w434:dbl)
        n288 = call "Interpolate RGB Color.vi"("Proportion"=w434, "Target Color"=u32 30976, "Base Color"=u32 2829099) -> ("Result Color"=w433:u32)  [unwired: 8 in]
      }
    }
    n289 = property class="Pane"(reference=w426, "PaneColor"=w425) -> ()  [unwired: 1 in, 2 out]
  }
  n290 = TCP Create Listener(10:u16 1741 ("timeout ms (25000)")) -> (3:w1:refnum<k5>)  [unwired: 4 in, 2 out]
  n291 = while {
    tunnel: w1 -> [w446]
    stop <- FALSE stop-if-true
    n292 = TCP Wait On Listener(11:w446) -> (4:w445:refnum<k5>)  [unwired: 3 in, 4 out]
    n293 = local write "TCP"(w445) -> ()
  }
  n294 = property on="On/Off" class="Bool (strict)"("Visible"=w6) -> ()  [unwired: 2 in, 2 out]
  n295 = property on="Motor" class="Clust (strict)"("Visible"=w6) -> ()  [unwired: 2 in, 2 out]
  n296 = property on="Progress" class="Clust (strict)"("Visible"=w6) -> ()  [unwired: 2 in, 2 out]
  n297 = property on="Test Ring" class="Ring (strict)"("Visible"=w6) -> ()  [unwired: 2 in, 2 out]
  n298 = property on="Rev/Fwd" class="Clust (strict)"("Visible"=w6) -> ()  [unwired: 2 in, 2 out]
  n299 = property on="Camera Settings" class="Clust (strict)"("Visible"=w6) -> ()  [unwired: 2 in, 2 out]
  n300 = local write "DB Camera Config"(w6) -> ()
  n301 = global write "WPI_DashboardLogging Global.vi" "Recording"(w32) -> ()
  n302 = local write "Rec Mode"(w32) -> ()
